vi "CopyFromScreen.vi"(8 "error in (no error)":errorcluster caption="错误输入（无错误）", 11 "Screen 输入":refnum<class "Screen.lvclass"> caption="DNL_LabVIEW Object in") -> (0 "error out":errorcluster caption="错误输出", 3 "Screen 输出":refnum<class "Screen.lvclass"> caption="DNL_LabVIEW Object out")   [LabVIEW 2011, in "Screen.lvclass"]
uses:
  Screen.lvclass
  Screen.lvclass/Screen.ctl
  System.Drawing
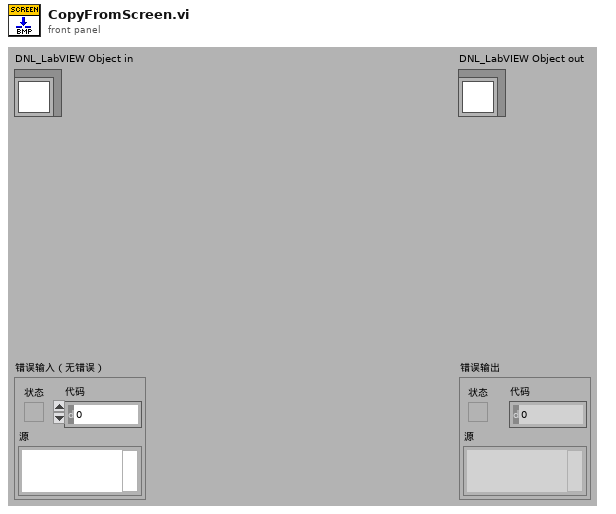
[diagram p1: front panel]
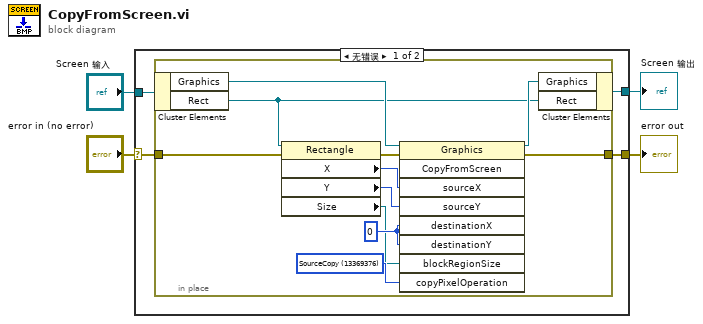
[diagram p0: block diagram]
diagram:
  n1 = case shown="无错误" "error in (no error)" {
    selector: "error in (no error)" -> [w7 w21]
    tunnel: [w6 w21] -> w3
    tunnel: [w5 w20] -> w1
    tunnel: "Screen 输入" -> [w8 w20]
    frame No Error {
      n2 = in-place {
        in-place-border: w7 -> [w11]
        in-place-border: [w10] -> w6
        w16 = 13369376 items=["Blackness"=66, "NotSourceErase"=1114278, "NotSourceCopy"=3342344, "SourceErase"=4457256, "DestinationInvert"=5570569, "PatInvert"=5898313, "SourceInvert"=6684742, "SourceAnd"=8913094, "MergePaint"=12255782, "MergeCopy"=12583114, "SourceCopy"=13369376, "SourcePaint"=15597702, "PatCopy"=15728673, "PatPaint"=16452105, "Whiteness"=16711778, "CaptureBlt"=1073741824, "NoMirrorBitmap"=-2147483648] ("copyPixelOperation")
        w17 = 0 ("destinationX")
        n3 = in-place-cluster #1(w8) -> ("Graphics"=w19:refnum<k24>, "Rect"=w9:refnum<k24>)
        n4 = property class="Rectangle"(reference=w9, error in=w11) -> (error out=w12:errorcluster, "X"=w14:i32, "Y"=w13:i32, "Size"=w15:refnum<k24>)  [unwired: 1 out]
        n5 = invoke class="Graphics" method="CopyFromScreen"(reference=w19, error in=w12, "sourceX"=w14, "sourceY"=w13, "destinationX"=w17, "destinationY"=w17, "blockRegionSize"=w15, "copyPixelOperation"=w16) -> (reference out=w18:refnum<k24>, error out=w10:errorcluster)  [unwired: 1 in, 7 out]
        n6 = in-place-cluster #1("Graphics"=w18, "Rect"=w9) -> (w5:refnum<class "Screen.lvclass">)
      }
    }
    frame Error {
    }
  }
  "error out" <- w3
  "Screen 输出" <- w1
